vi "rad_Deploy Images with Progress_FB.vi"(6 "Deployment Notifiers":T1[](array[typedef]), 7 "temp folder":path, 8 "error in (no error)":errorcluster, 9 "Target Config Options in":T4={"NumInBatch"=0, "Target Config Operation"=enum."No Config", "Target Name"="", "Increment Static IPs"=FALSE, "Change Target Name"=FALSE, "Primary NIC"={"MAC address"="", "IP Address Request Mode"=2, "IP address"="", "Subnet mask"="", "Gateway"="", "DNS server"=""}} {"Primary NIC"."IP Address Request Mode" items=["Static"=1, "DHCP/Link-Local"=2, "Link-Local Only"=4, "DHCP Only"=8]}, 10 "RT Deployment Targets in":T2[](array[typedef]) {"Primary NIC"."IP Address Request Mode" items=["Static"=1, "DHCP/Link-Local"=2, "Link-Local Only"=4, "DHCP Only"=8]}, 11 "image path":path) -> (0 "error out":errorcluster, 1 "Target Config Options out":T4={"NumInBatch"=0, "Target Config Operation"=enum."No Config", "Target Name"="", "Increment Static IPs"=FALSE, "Change Target Name"=FALSE, "Primary NIC"={"MAC address"="", "IP Address Request Mode"=2, "IP address"="", "Subnet mask"="", "Gateway"="", "DNS server"=""}} {"Primary NIC"."IP Address Request Mode" items=["Static"=1, "DHCP/Link-Local"=2, "Link-Local Only"=4, "DHCP Only"=8]}, 2 "Error Occurred":bool[](array[boolean]))   [LabVIEW 2015]
uses:
  TypeDefs/rad_Target Configuration Settings.ctl
  TypeDefs/rad_Target Configuration Operations.ctl
  Targets/TypeDefs/rad_Target Network Settings.ctl
  Targets/TypeDefs/rad_Target Information.ctl
  TypeDefs/rad_Application Image Properties.ctl
  TypeDefs/rad_FPGA Properties.ctl
  TypeDefs/rad_FPGA Flash Properties.ctl
  TypeDefs/rad_Deployment Notifiers.ctl
  TypeDefs/rad_Deployment Status Data Type.ctl
  TypeDefs/rad_Deployment Progress Data Type.ctl
  Targets/TypeDefs/rad_Initialize Access Types.ctl
  <vilib>/nisyscfg/Close (System).vi
  <vilib>/nisyscfg/Set System Image (Folder).vi
  <vilib>/nisyscfg/nisyscfg.lvlib
panel:
  out "AppImage Properties.Model":string
  in  "State Variables":T10={"INI Modified"=FALSE, "Target Config. Options"={"NumInBatch"=0, "Target Config Operation"=enum."No Config", "Target Name"="", "Increment Static IPs"=FALSE, "Change Target Name"=FALSE, "Primary NIC"={"MAC address"="", "IP Address Request Mode"=2, "IP address"="", "Subnet mask"="", "Gateway"="", "DNS server"=""}}, "RT Deployment Targets"=[], "AppImage Properties"={"Name"="", "Version"="", "Time"=timestamp(0 s since 1904-01-01), "Description"="", "Key"="", "Chassis"="", "FPGA Properties"=[], "Model"="", "Retrieve"=[], "Deploy"=[], "Installed Software"=[]}, "Deployment Notifiers"=[], "Post-deployment access"=enum."Admin unless unlocked"} {"RT Deployment Targets"."Primary NIC"."IP Address Request Mode" items=["Static"=1, "DHCP/Link-Local"=2, "Link-Local Only"=4, "DHCP Only"=8]; "Target Config. Options"."Primary NIC"."IP Address Request Mode" items=["Static"=1, "DHCP/Link-Local"=2, "Link-Local Only"=4, "DHCP Only"=8]}
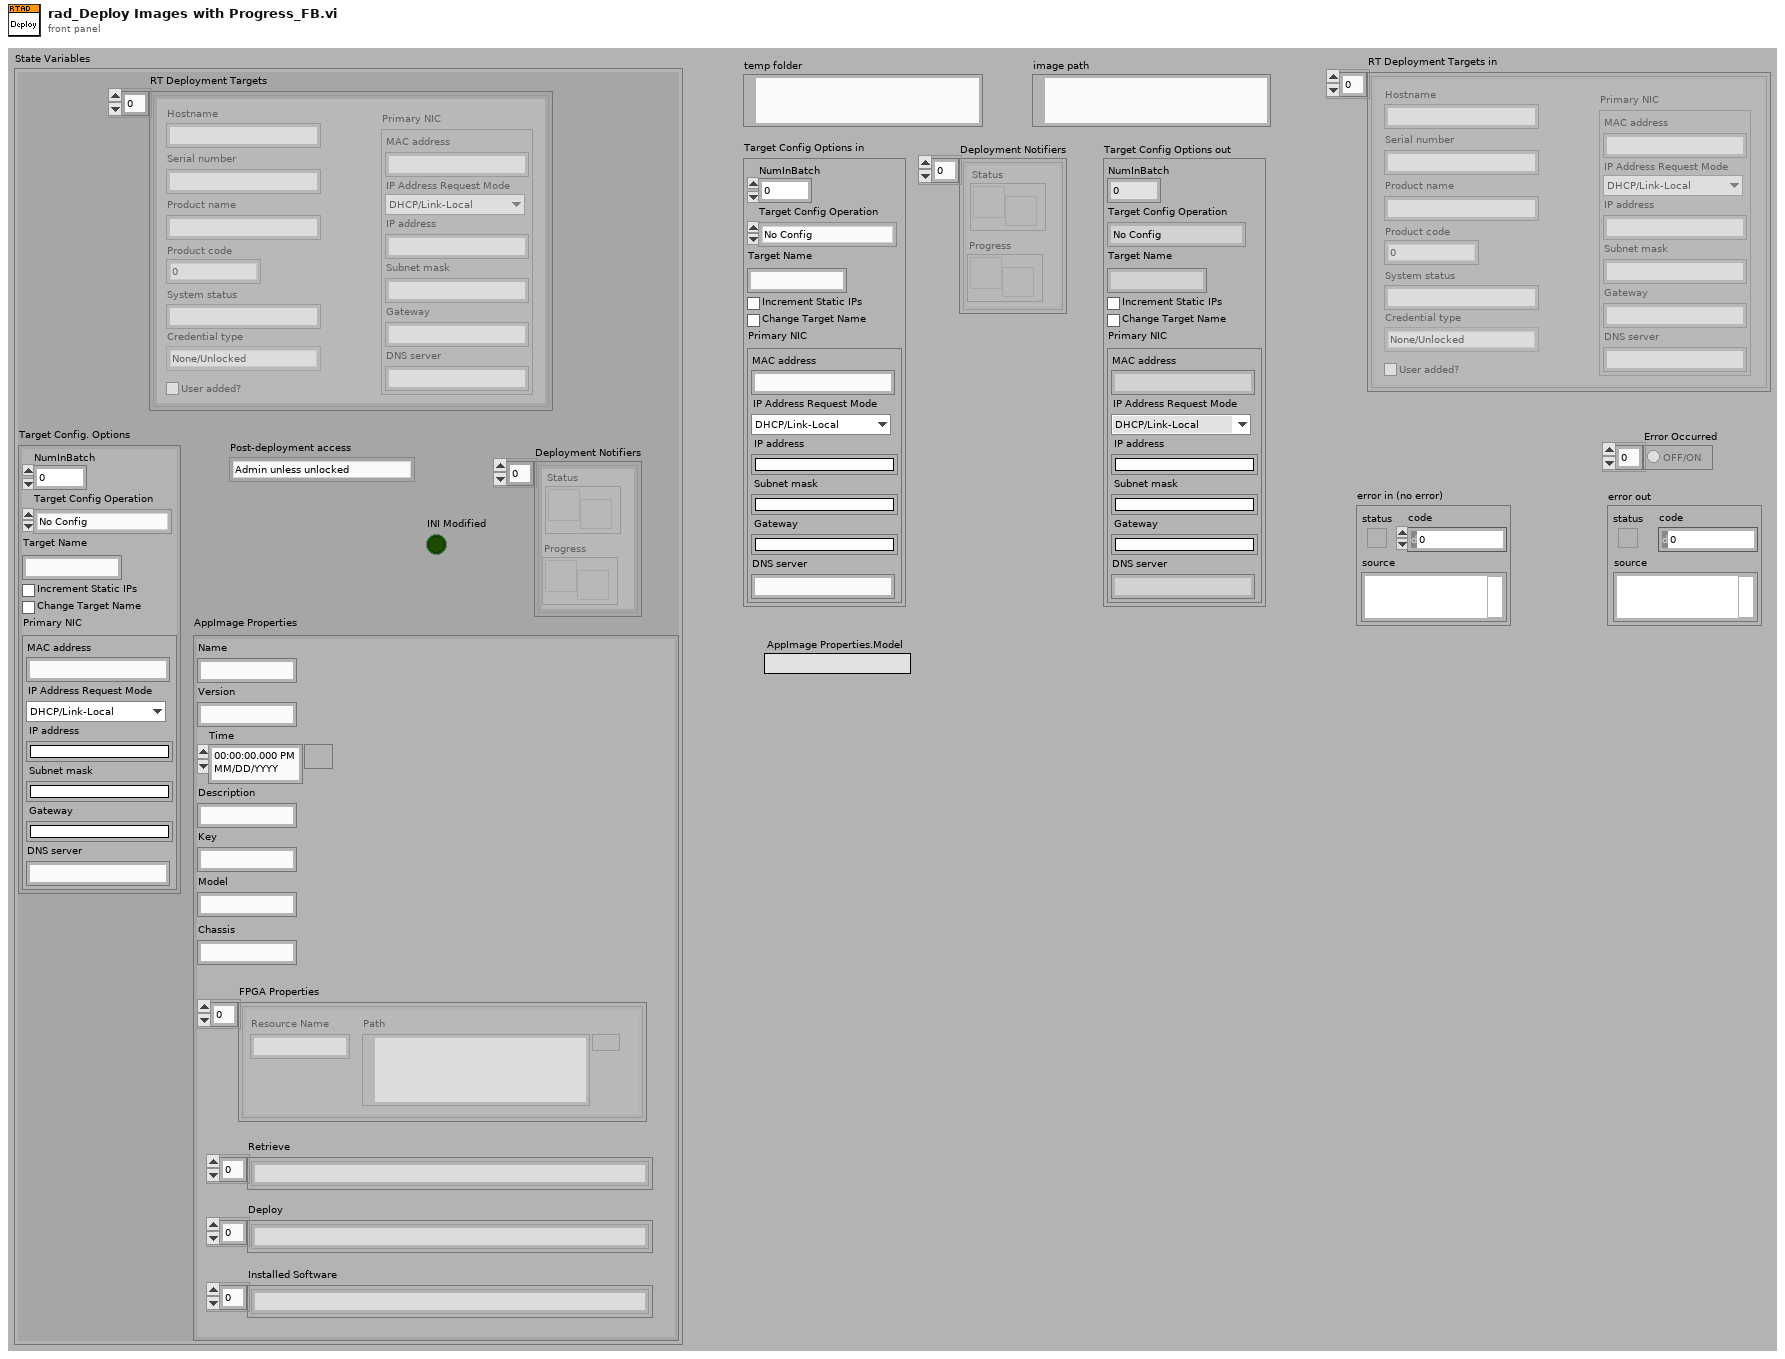
[diagram p1: front panel]
types:
  T1 = typedef "rad_Deployment Notifiers.ctl" = cluster{"Status":refnum<notifier>, "Progress":refnum<notifier>}
  T2 = typedef "rad_Target Information.ctl" = cluster{"Hostname":string, "Serial number":string, "Product name":string, "Product code":i32, "System status":string, "Credential type":enum16{"None/Unlocked", "FTP Password", "NIAuth Credentials"}, "User added?":bool, "Primary NIC":T3}
  T3 = typedef "rad_Target Network Settings.ctl" = cluster{"MAC address":string, "IP Address Request Mode":i32, "IP address":string, "Subnet mask":string, "Gateway":string, "DNS server":string}
  T4 = typedef "rad_Target Configuration Settings.ctl" = cluster{"NumInBatch":u32, "Target Config Operation":T5, "Target Name":string, "Increment Static IPs":bool, "Change Target Name":bool, "Primary NIC":T3}
  T5 = typedef "rad_Target Configuration Operations.ctl" = enum8{"No Config", "Image Config", "Static Config"}
  T6 = typedef "rad_Application Image Properties.ctl" = cluster{"Name":string, "Version":string, "Time":timestamp, "Description":string, "Key":string, "Chassis":string, "FPGA Properties":T7, "Model":string, "Retrieve":string[], "Deploy":string[], "Installed Software":string[]}
  T7 = typedef "rad_FPGA Properties.ctl" = T8[]
  T8 = typedef "rad_FPGA Flash Properties.ctl" = cluster{"Resource Name":string, "Path":path}
  T9 = typedef "rad_Initialize Access Types.ctl" = enum16{"Anonymous read-only", "Admin unless unlocked", "Admin always"}
  T10 = cluster{"INI Modified":bool, "Target Config. Options":T4, "RT Deployment Targets":T2[], "AppImage Properties":T6, "Deployment Notifiers":T1[], "Post-deployment access":T9}
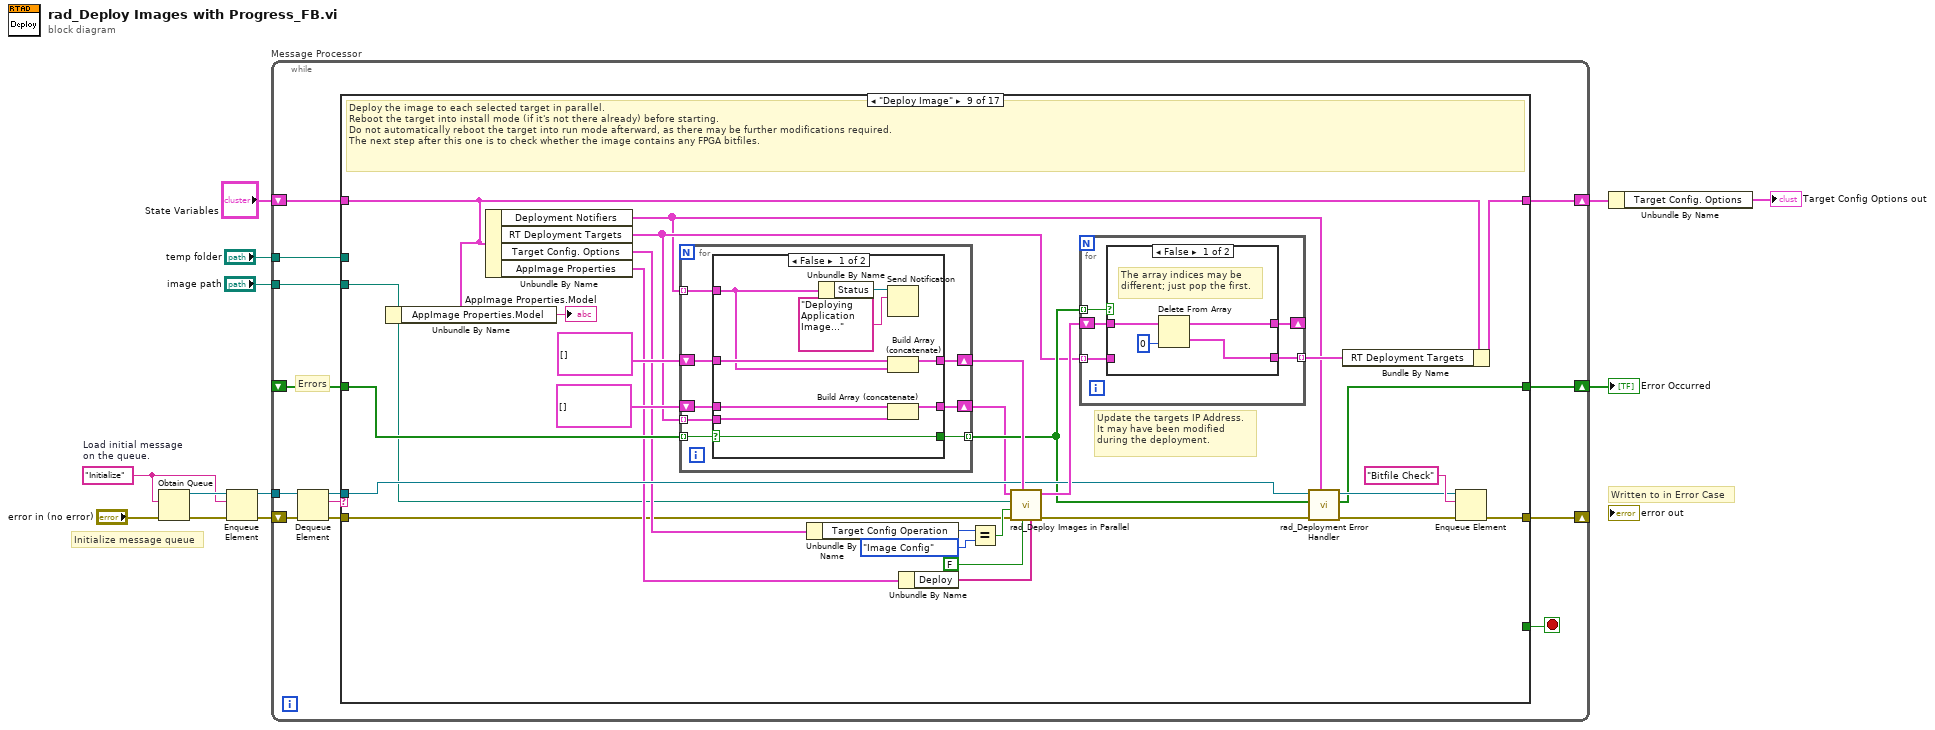
[diagram p0: block diagram]
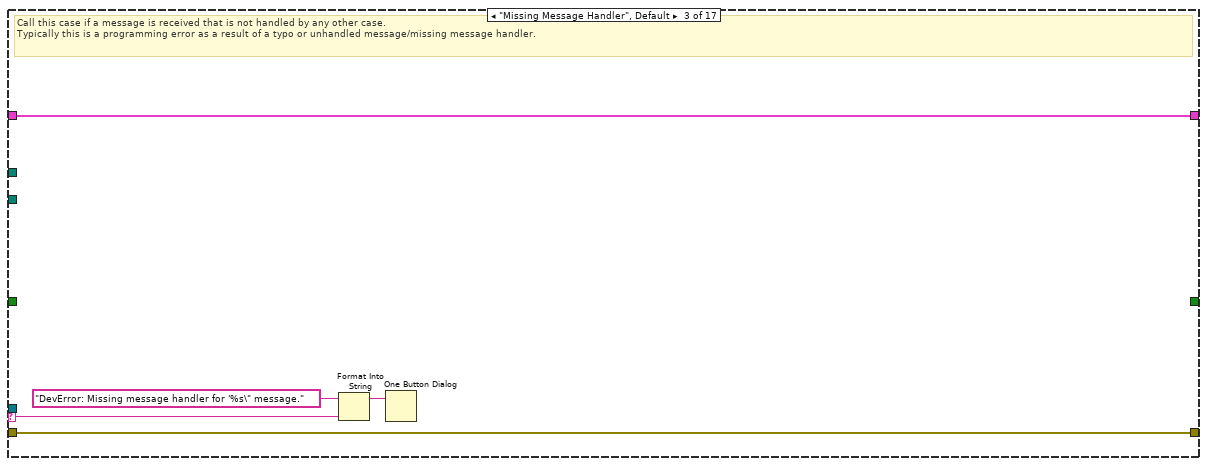
[diagram p4: hidden frame]
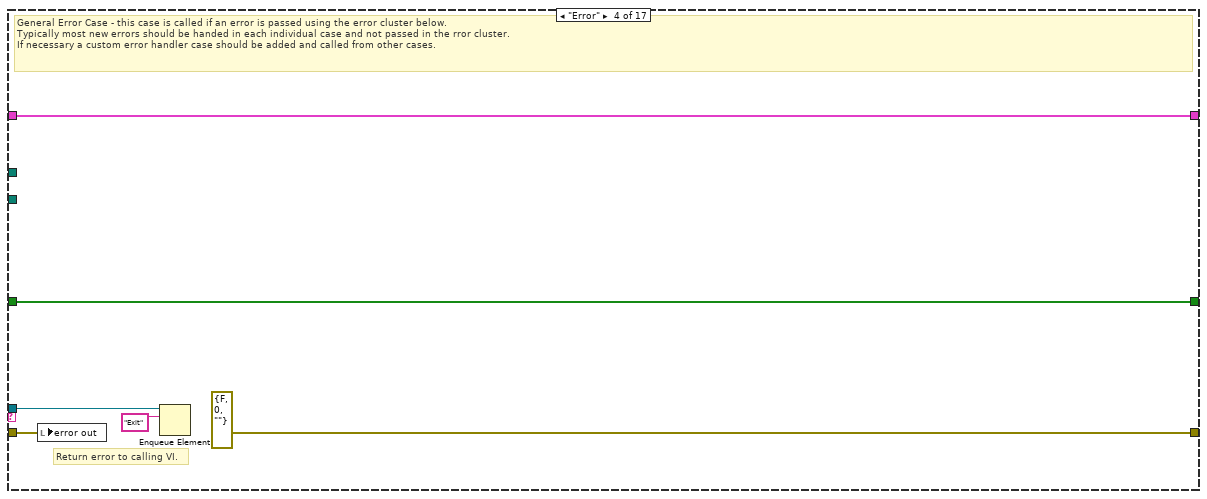
[diagram p5: hidden frame]
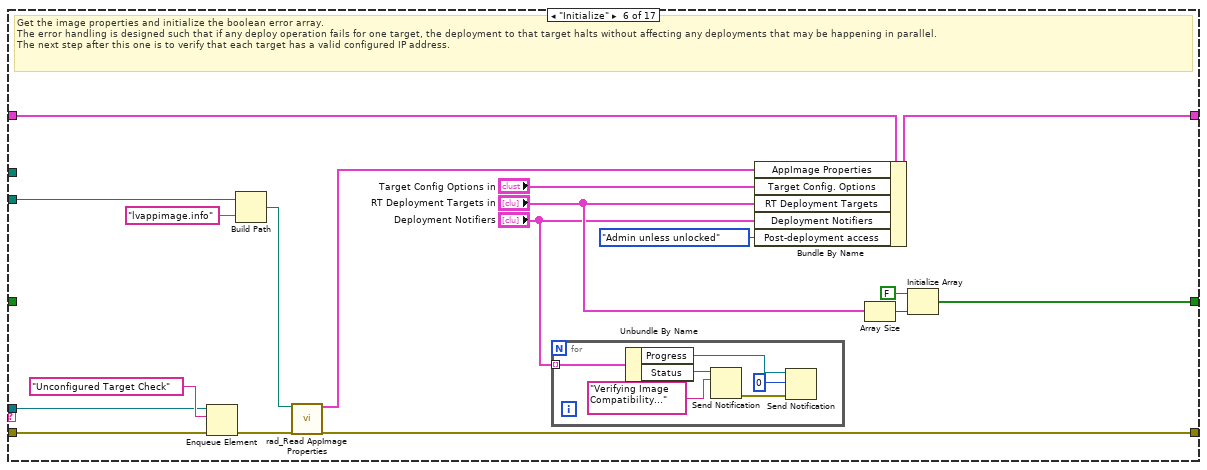
[diagram p7: hidden frame]
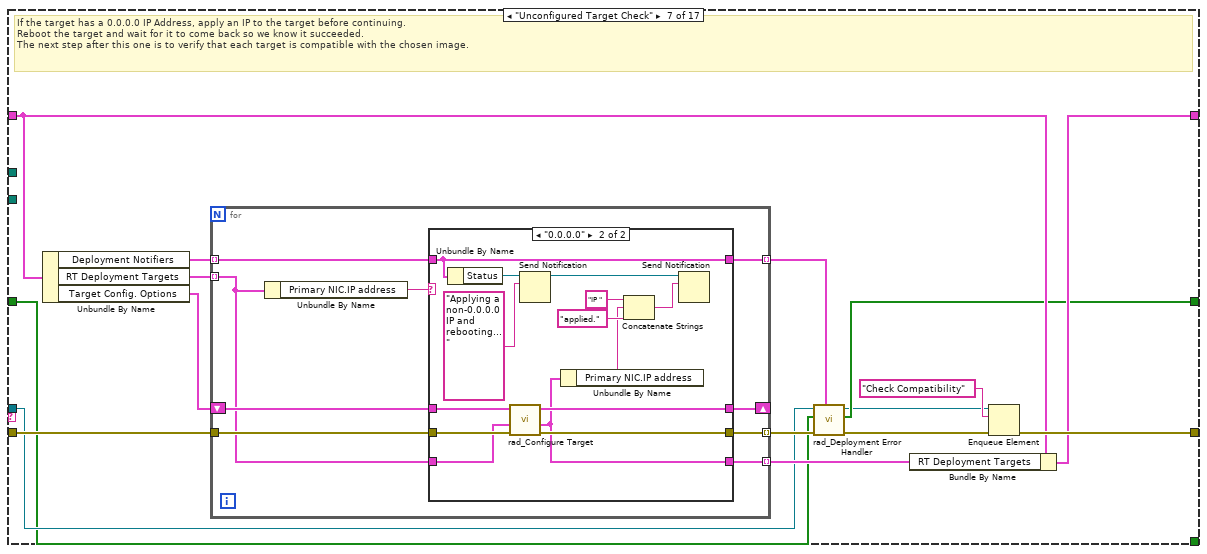
[diagram p8: hidden frame]
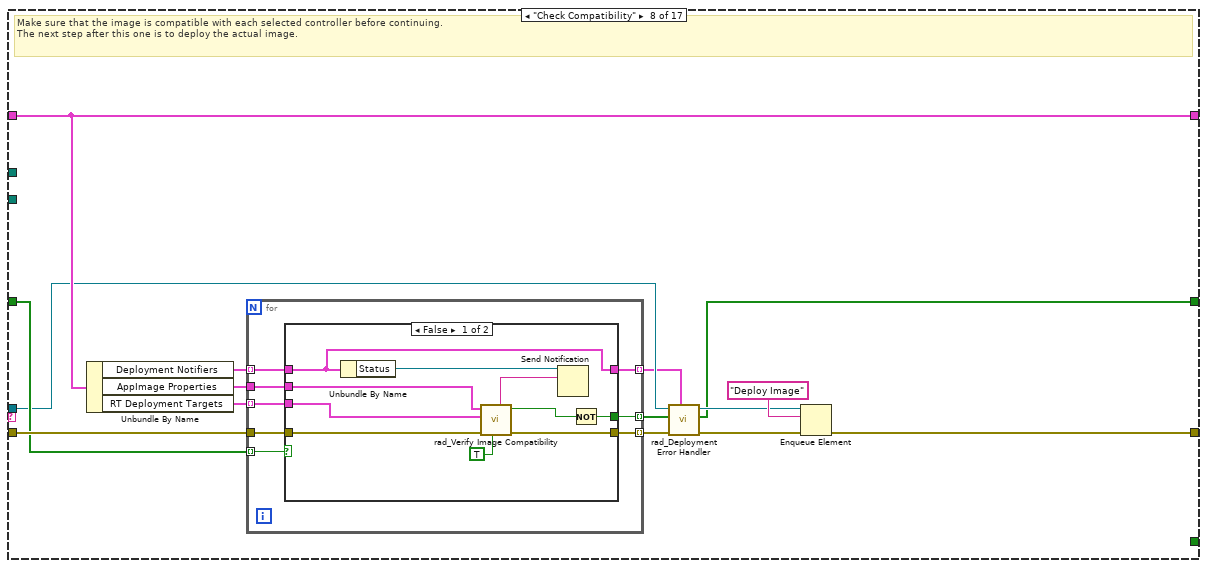
[diagram p10: hidden frame]
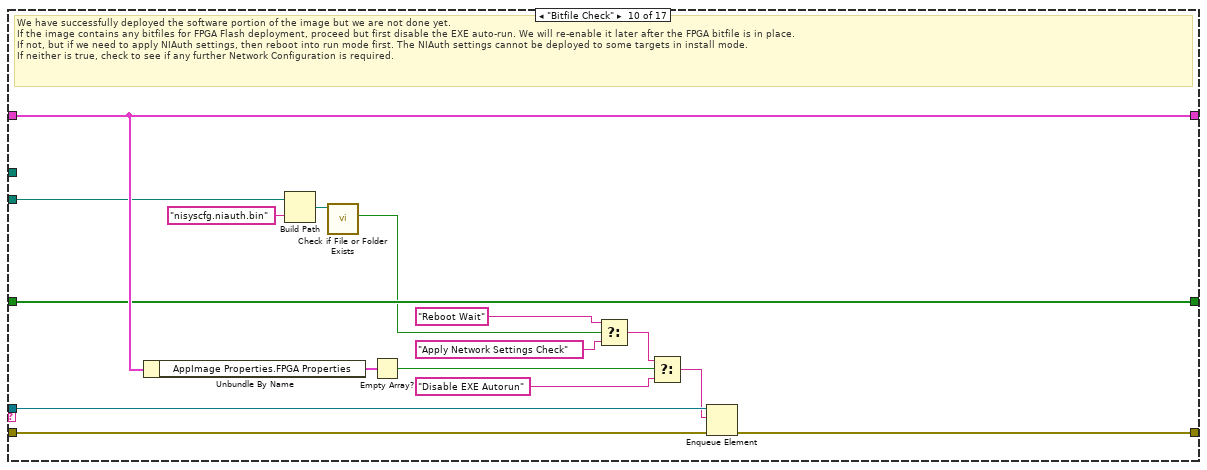
[diagram p14: hidden frame]
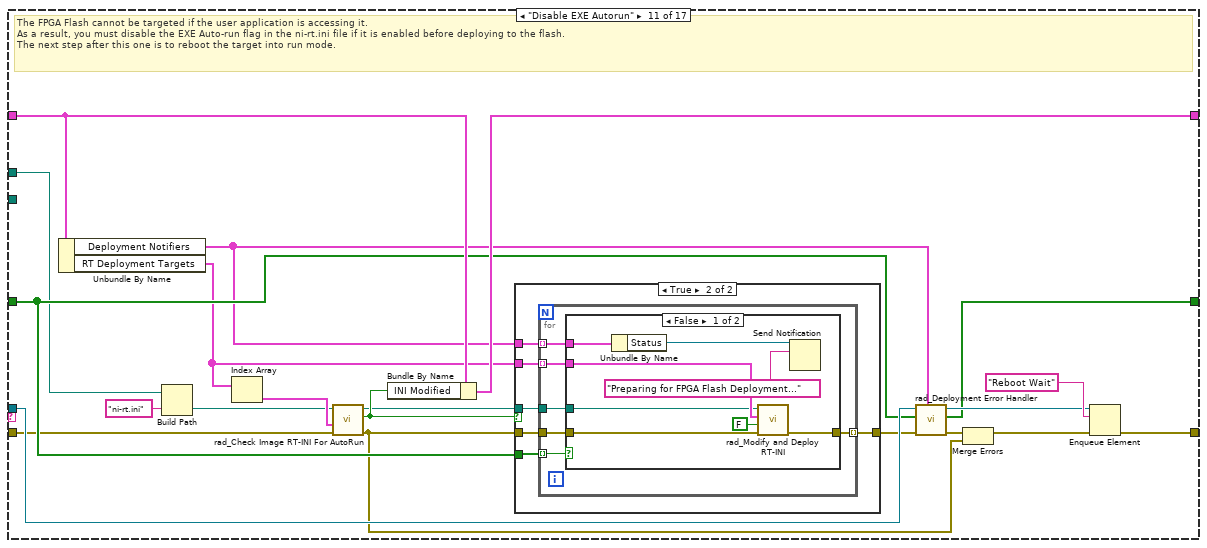
[diagram p15: hidden frame]
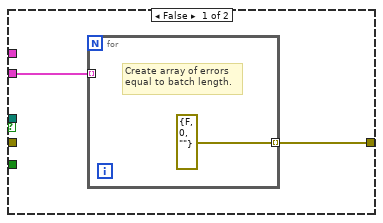
[diagram p16: hidden frame]
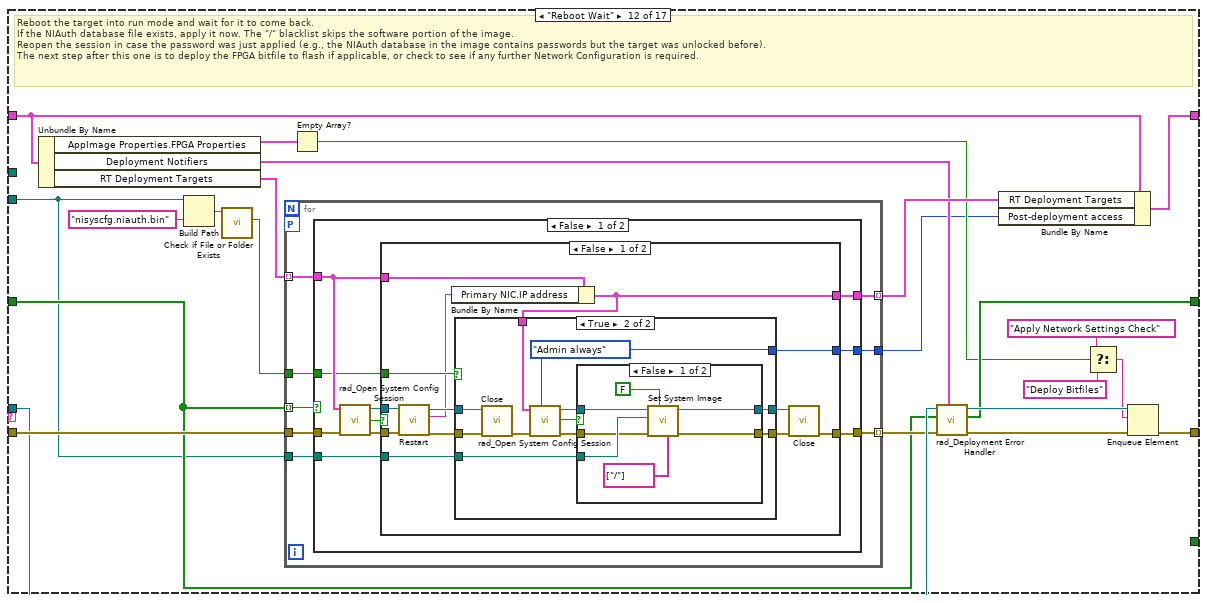
[diagram p18: hidden frame]
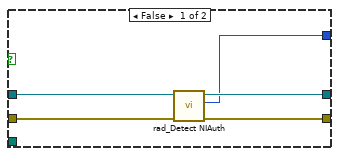
[diagram p19: hidden frame]
diagram:
  w1 = "Initialize"  # Load initial message on the queue.
  # "Written to in Error Case"
  # "Initialize message queue"
  n1 = Obtain Queue(element data type=w1, error in (no error)="error in (no error)") -> (queue out=w12:refnum<queue>, error out=w3:errorcluster)  [unwired: 3 in, 1 out]
  n2 = Enqueue Element(queue=w12, element=w1, error in (no error)=w3) -> (queue out=w4:refnum<queue>, error out=w2:errorcluster)  [unwired: 1 in, 1 out]
  n3 = while "Message Processor" {
    shift-left: w2 -> [w21]
    shift-right: [w14] -> _
    tunnel: w4 -> [w22]
    shift-left: "State Variables" -> [w25]
    shift-right: [w24] -> w9
    tunnel: "temp folder" -> [w18]
    tunnel: "image path" -> [w17]
    shift-right: [w15] -> w5
    shift-left: _ -> [w16]
    stop <- w13 stop-if-true
    # "Errors"
    n4 = Dequeue Element(queue=w22, error in (no error)=w21) -> (queue out=w23:refnum<queue>, element=w19:string, error out=w20:errorcluster)  [unwired: 1 in, 1 out]
    n5 = case shown="\"Deploy Image\"" w19 {
      selector: w19 -> [_ _ w33 _ _ _ _ _ _ _ _ _ _ _ _ _ _]
      tunnel: [w27 w30 w35 w41 w43 w60 w80 w124 w168 w220 w240 w285 w373 w413 w442 w489 w513] -> w24
      tunnel: w25 -> [w27 w30 w35 w41 w43 w61 w79 w124 w148 w220 w241 w287 w373 w413 w440 w489 w513]
      tunnel: w23 -> [_ _ _ w40 _ w45 w70 w117 w166 w221 w239 w283 w367 w410 w433 w496 w515]
      tunnel: w20 -> [w26 w29 w34 w37 w42 w50 w83 w119 w149 w219 w225 w288 w356 w401 w441 w498 w516]
      tunnel: [w26 w29 w34 errorcluster {"status"=FALSE, "code"=0, "source"=""} ("error out") w42 w51 w82 w125 w175 w222 w243 w290 w374 w412 w446 w500 w514] -> w14
      tunnel: w18 -> [_ _ _ _ _ _ _ _ _ _ w226 _ _ w402 _ _ _]
      tunnel: w17 -> [_ _ _ _ _ w49 _ _ w150 w214 _ w273 w355 _ _ _ _]
      tunnel: [_ w28 _ w36 _ w56 w74 w112 w161 w218 w236 w281 w366 w408 w431 w494 w511] -> w15
      tunnel: w16 -> [_ w28 _ w36 _ _ w68 w118 w173 w218 w233 w278 w362 w406 w426 w491 w511]
      tunnel: [_ _ _ _ _ _ _ _ _ _ _ _ _ _ _ _ TRUE] -> w13
      frame "---------- Framework Operations ----------" {
        # "Dummy case to add a seperator in the Case Structure menu."
      }
      frame "", "Idle" {
        # "Idle Case - this case is called after a Timeout on the Get Next Message from Queue VI, if no new messages are present on the queue.\nThis case can be used for housekeeping tasks such as updating the UI."
      }
      frame "Missing Message Handler", Default {
        # "Call this case if a message is received that is not handled by any other case.\nTypically this is a programming error as a result of a typo or unhandled message/missing message handler."
        n6 = Format Into String(format string="DevError: Missing message handler for '%s\" message." ("message"), w33) -> (resulting string=w31:string)  [unwired: 2 in, 1 out]
        n7 = One Button Dialog(message=w31) -> ()  [unwired: 2 out]
      }
      frame "Error" {
        # "Return error to calling VI."
        # "General Error Case - this case is called if an error is passed using the error cluster below.\nTypically most new errors should be handed in each individual case and not passed in the rror cluster.\nIf necessary a custom error handler case should be added and called from other cases."
        n8 = local write "error out"(w37) -> ()
        n9 = Enqueue Element(queue=w40, element="Exit") -> ()  [unwired: 2 in, 3 out]
      }
      frame "----------Application Operations ----------" {
        # "Dummy case to add a seperator in the Case Structure menu."
      }
      frame "Initialize" {
        # "Get the image properties and initialize the boolean error array. \nThe error handling is designed such that if any deploy operation fails for one target, the deployment to that target halts without affecting any deployments that may be happening in parallel. \nThe next step after this one is to verify that each target has a valid configured IP address."
        n10 = Enqueue Element(queue=w45, element="Unconfigured Target Check", error in (no error)=w50) -> (error out=w47:errorcluster)  [unwired: 1 in, 2 out]
        n11 = Build Path(base path=w49, name or relative path="lvappimage.info") -> (appended path=w52:path)
        n12 = call "rad_Read AppImage Properties.vi"("AppImage Properties Path"=w52, "error in (no error)"=w47) -> ("AppImage Properties"=w48:T6, "error out"=w51:errorcluster)  [unwired: 12 in, 4 out]
        n13 = for {
          tunnel: "Deployment Notifiers" -> [w66] mode=indexing
          n14 = Unbundle By Name(w66) -> ("Progress"=w64:refnum<notifier>, "Status"=w65:refnum<notifier>)
          n15 = Send Notification(notification="Verifying Image Compatibility...", notifier=w65) -> (error out=w63:errorcluster)  [unwired: 1 in, 1 out]
          n16 = Send Notification(notification=0, notifier=w64, error in (no error)=w63) -> ()  [unwired: 2 out]
        }
        n17 = Bundle By Name(cluster=w61, "AppImage Properties"=w48, "Target Config. Options"="Target Config Options in", "RT Deployment Targets"="RT Deployment Targets in", "Deployment Notifiers"="Deployment Notifiers", "Post-deployment access"=rad_Initialize_Access_Types."Admin unless unlocked") -> (w60:T10)
        n18 = Array Size(array="RT Deployment Targets in") -> (size(s)=w57:i32)
        n19 = Initialize Array(FALSE, w57) -> (w56:bool[])
      }
      frame "Unconfigured Target Check" {
        # "If the target has a 0.0.0.0 IP Address, apply an IP to the target before continuing. \nReboot the target and wait for it to come back so we know it succeeded. \nThe next step after this one is to verify that each target is compatible with the chosen image."
        n20 = Unbundle By Name(w79) -> ("Deployment Notifiers"=w78:T1[], "RT Deployment Targets"=w77:T2[], "Target Config. Options"=w76:T4)
        n21 = for {
          tunnel: w83 -> [w90]
          tunnel: [w92] -> w73 mode=indexing
          tunnel: w78 -> [w88] mode=indexing
          tunnel: w77 -> [w87] mode=indexing
          shift-right: [w89] -> _
          shift-left: w76 -> [w91]
          tunnel: [w86] -> w75 mode=indexing
          tunnel: [w85] -> w71 mode=indexing
          n22 = Unbundle By Name(w87) -> ("Primary NIC.IP address"=w84:string)
          n23 = case shown="\"0.0.0.0\"" w84 {
            tunnel: [w96 w102] -> w92
            tunnel: w91 -> [w94 w110]
            tunnel: w90 -> [w96 w103]
            tunnel: [w94 w109] -> w89
            tunnel: w88 -> [w93 w100]
            tunnel: w87 -> [w95 w99]
            tunnel: [w95 w98] -> w86
            tunnel: [w93 w100] -> w85
            frame Default {
            }
            frame "0.0.0.0" {
              n24 = Unbundle By Name(w100) -> ("Status"=w101:refnum<notifier>)
              n25 = call "rad_Configure Target.vi"("error in (no error)"=w103, "Target settings in"=w99, "Target Config Options in"=w110) -> ("error out"=w102:errorcluster, "Target settings out"=w98:T2, "Target Config Options out"=w109:T4)  [unwired: 6 in]
              n26 = Send Notification(notification="Applying a non-0.0.0.0 IP and rebooting...", notifier=w101) -> (notifier out=w107:refnum<notifier>)  [unwired: 1 in, 1 out]
              n27 = Unbundle By Name(w98) -> ("Primary NIC.IP address"=w97:string)
              n28 = Concatenate Strings("IP " ("notification"), w97, "applied." ("string")) -> (w104:string)
              n29 = Send Notification(notification=w104, notifier=w107) -> ()  [unwired: 1 in, 2 out]
            }
          }
        }
        n30 = call "rad_Deployment Error Handler.vi"("Deployment Notifiers"=w71, "error in (no error)"=w73, "Error Occurred"=w68, "Queue in"=w70) -> ("error out"=w72:errorcluster, "Error Occurred"=w74:bool[], "Queue out"=w69:refnum<queue>)  [unwired: 5 in]
        n31 = Bundle By Name(cluster=w79, "RT Deployment Targets"=w75) -> (w80:T10)
        n32 = Enqueue Element(queue=w69, element="Check Compatibility" ("Message Name"), error in (no error)=w72) -> (error out=w82:errorcluster)  [unwired: 1 in, 2 out]
      }
      frame "Check Compatibility" {
        # "Make sure that the image is compatible with each selected controller before continuing.\nThe next step after this one is to deploy the actual image."
        n33 = Unbundle By Name(w124) -> ("Deployment Notifiers"=w121:T1[], "AppImage Properties"=w120:T6, "RT Deployment Targets"=w122:T2[])
        n34 = for {
          tunnel: w122 -> [w131] mode=indexing
          tunnel: w121 -> [w129] mode=indexing
          tunnel: w120 -> [w133]
          tunnel: w119 -> [w132]
          tunnel: w118 -> [w130] mode=indexing
          tunnel: [w128] -> w115 mode=indexing
          tunnel: [w127] -> w116 mode=indexing
          tunnel: [w126] -> w114 mode=indexing
          n35 = case shown="False" w130 {
            selector: w130 -> [_ w146]
            tunnel: w133 -> [w143 _]
            tunnel: w132 -> [w142 w145]
            tunnel: w131 -> [w134 _]
            tunnel: w129 -> [w136 w144]
            tunnel: [w138 w146] -> w128
            tunnel: [w140 w145] -> w127
            tunnel: [w136 w144] -> w126
            frame False {
              n36 = Unbundle By Name(w136) -> ("Status"=w137:refnum<notifier>)
              n37 = call "rad_Verify Image Compatibility.vi"("Require Identical Chassis?"=TRUE, "error in (no error)"=w142, "Target address"=w134, "AppImage Properties"=w143) -> ("error out"=w140:errorcluster, "Compatible?"=w139:bool, "Status message"=w135:string)  [unwired: 5 in]
              n38 = Send Notification(notification=w135, notifier=w137) -> ()  [unwired: 1 in, 2 out]
              n39 = Not(x=w139) -> (.not. x?=w138:bool)
            }
            frame True {
            }
          }
        }
        n40 = call "rad_Deployment Error Handler.vi"("Deployment Notifiers"=w114, "error in (no error)"=w116, "Error Occurred"=w115, "Queue in"=w117) -> ("error out"=w111:errorcluster, "Error Occurred"=w112:bool[], "Queue out"=w113:refnum<queue>)  [unwired: 5 in]
        n41 = Enqueue Element(queue=w113, element="Deploy Image" ("t"), error in (no error)=w111) -> (error out=w125:errorcluster)  [unwired: 1 in, 2 out]
      }
      frame "Deploy Image" {
        # "Update the targets IP Address.\nIt may have been modified\nduring the deployment."
        # "Deploy the image to each selected target in parallel. \nReboot the target into install mode (if it's not there already) before starting.\nDo not automatically reboot the target into run mode afterward, as there may be further modifications required. \nThe next step after this one is to check whether the image contains any FPGA bitfiles."
        n42 = Unbundle By Name(w148) -> ("AppImage Properties.Model"=→"AppImage Properties.Model":string)
        n43 = Unbundle By Name(w148) -> ("Deployment Notifiers"=w158:T1[], "RT Deployment Targets"=w159:T2[], "Target Config. Options"=w154:T4, "AppImage Properties"=w153:T6)
        n44 = for {
          tunnel: w158 -> [w193] mode=indexing
          tunnel: w173 -> [w194] mode=indexing
          tunnel: [w192] -> w164 mode=indexing
          tunnel: w159 -> [w191] mode=indexing
          shift-right: [w190] -> w170
          shift-left: T1[] [] ("Deployment Notifiers") -> [w189]
          shift-right: [w188] -> w151
          shift-left: T2[] [] -> [w187]
          n45 = case shown="False" w194 {
            selector: w194 -> [w202 w206]
            tunnel: w193 -> [w197 _]
            tunnel: [w202 w206] -> w192
            tunnel: w191 -> [w195 _]
            tunnel: [w201 w204] -> w190
            tunnel: w189 -> [w200 w204]
            tunnel: [w199 w205] -> w188
            tunnel: w187 -> [w198 w205]
            frame False {
              n46 = Unbundle By Name(w197) -> ("Status"=w196:refnum<notifier>)
              n47 = Send Notification(notification="Deploying Application Image...", notifier=w196) -> ()  [unwired: 1 in, 2 out]
              n48 = Build Array (concatenate)(w200, w197) -> (w201:T1[])
              n49 = Build Array (concatenate)(w198, w195) -> (w199:T2[])
            }
            frame True {
            }
          }
        }
        n50 = Unbundle By Name(w154) -> ("Target Config Operation"=w157:T5)
        n51 = Unbundle By Name(w153) -> ("Deploy"=w152:string[])
        n52 = Equal?(x=w157, y=rad_Target_Configuration_Operations."Image Config" ("x")) -> (x = y?=w155:bool)
        n53 = call "rad_Deploy Images in Parallel.vi"("Deploy"=w152, "restart after imaging (T)"=FALSE ("restart after imaging? (T)"), "Deployment Notifiers"=w170, "error in (no error)"=w149, "apply primary NIC from image (F)"=w155, "image file path in"=w150, "Target addresses in"=w151) -> ("Errors Out"=w165:errorcluster[], "Target addresses out"=w169:T2[])  [unwired: 2 in, 1 out]
        n54 = for {
          tunnel: w164 -> [w180] mode=indexing
          tunnel: w159 -> [w178] mode=indexing
          shift-right: [w176] -> _
          shift-left: w169 -> [w179]
          tunnel: [w177] -> w167 mode=indexing
          n55 = case shown="False" w180 {
            tunnel: w179 -> [w184 w186]
            tunnel: w178 -> [_ w185]
            tunnel: [w182 w185] -> w177
            tunnel: [w183 w186] -> w176
            frame False {
              # "The array indices may be\ndifferent; just pop the first."
              n56 = Delete From Array(array=w184, index=0) -> (deleted portion=w182:T2, array with subset deleted=w183:T2[])  [unwired: 1 in]
            }
            frame True {
              # "An error happened earlier,\nso keep the existing address."
            }
          }
        }
        n57 = call "rad_Deployment Error Handler.vi"("Deployment Notifiers"=w158, "error in (no error)"=w165, "Error Occurred"=w164, "Queue in"=w166) -> ("error out"=w162:errorcluster, "Error Occurred"=w161:bool[], "Queue out"=w163:refnum<queue>)  [unwired: 5 in]
        n58 = Bundle By Name(cluster=w148, "RT Deployment Targets"=w167) -> (w168:T10)
        n59 = Enqueue Element(queue=w163, element="Bitfile Check" ("Message Name"), error in (no error)=w162) -> (error out=w175:errorcluster)  [unwired: 1 in, 2 out]
      }
      frame "Bitfile Check" {
        # "We have successfully deployed the software portion of the image but we are not done yet.\nIf the image contains any bitfiles for FPGA Flash deployment, proceed but first disable the EXE auto-run. We will re-enable it later after the FPGA bitfile is in place.\nIf not, but if we need to apply NIAuth settings, then reboot into run mode first. The NIAuth settings cannot be deployed to some targets in install mode.\nIf neither is true, check to see if any further Network Configuration is required."
        n60 = Unbundle By Name(w220) -> ("AppImage Properties.FPGA Properties"=w217:T7)
        n61 = Build Path(base path=w214, name or relative path="nisyscfg.niauth.bin") -> (appended path=w212:path)
        n62 = call <vilib>:"Check if File or Folder Exists.vi"("path"=w212) -> ("file or folder exists?"=w209:bool)  [unwired: 8 in, 2 out]
        n63 = Empty Array?(array=w217) -> (empty?=w215:bool)
        n64 = Select(t="Reboot Wait" ("Title"), s=w209, f="Apply Network Settings Check" ("Title")) -> (s? t:f=w210:string)
        n65 = Select(t=w210, s=w215, f="Disable EXE Autorun" ("Title")) -> (s? t:f=w211:string)
        n66 = Enqueue Element(queue=w221, element=w211, error in (no error)=w219) -> (error out=w222:errorcluster)  [unwired: 1 in, 2 out]
      }
      frame "Disable EXE Autorun" {
        # "The FPGA Flash cannot be targeted if the user application is accessing it.\nAs a result, you must disable the EXE Auto-run flag in the ni-rt.ini file if it is enabled before deploying to the flash.\nThe next step after this one is to reboot the target into run mode."
        n67 = Unbundle By Name(w241) -> ("Deployment Notifiers"=w232:T1[], "RT Deployment Targets"=w231:T2[])
        n68 = Build Path(base path=w226, name or relative path="ni-rt.ini") -> (appended path=w224:path)
        n69 = Index Array(array=w231) -> (element=w227:T2)  [unwired: 1 in]
        n70 = call "rad_Check Image RT-INI For AutoRun.vi"("error in (no error)"=w225, "target settings"=w227, "temp folder"=w224) -> ("error out"=w230:errorcluster, "Run at Startup?"=w229:bool, "temp folder out"=w228:path)  [unwired: 6 in]
        n71 = Bundle By Name(cluster=w241, "INI Modified"=w229) -> (w240:T10)
        n72 = case shown="True" w229 {
          tunnel: [w244 w251] -> w237
          tunnel: w230 -> [_ w252]
          tunnel: w231 -> [w245 w250]
          tunnel: w233 -> [_ w249]
          tunnel: w232 -> [_ w248]
          tunnel: w228 -> [_ w247]
          frame False {
            n73 = for {
              tunnel: w245 -> [_] mode=indexing
              tunnel: [errorcluster {"status"=FALSE, "code"=0, "source"=""} ("error out")] -> w244 mode=indexing
              # "Create array of errors\nequal to batch length."
            }
          }
          frame True {
            n74 = for {
              tunnel: w252 -> [w258]
              tunnel: [w257] -> w251 mode=indexing
              tunnel: w250 -> [w256] mode=indexing
              tunnel: w249 -> [w255] mode=indexing
              tunnel: w248 -> [w254] mode=indexing
              tunnel: w247 -> [w253]
              n75 = case shown="False" w255 {
                tunnel: w258 -> [w260 w267]
                tunnel: [w265 w267] -> w257
                tunnel: w256 -> [w261 _]
                tunnel: w254 -> [w263 _]
                tunnel: w253 -> [w259 _]
                frame False {
                  n76 = Unbundle By Name(w263) -> ("Status"=w262:refnum<notifier>)
                  n77 = call "rad_Modify and Deploy RT-INI.vi"("error in (no error)"=w260, "Run at Startup?"=FALSE, "Target settings"=w261, "temp folder"=w259) -> ("error out"=w265:errorcluster)  [unwired: 7 in]
                  n78 = Send Notification(notification="Preparing for FPGA Flash Deployment...", notifier=w262) -> ()  [unwired: 1 in, 2 out]
                }
                frame True {
                }
              }
            }
          }
        }
        n79 = call "rad_Deployment Error Handler.vi"("Deployment Notifiers"=w232, "error in (no error)"=w237, "Error Occurred"=w233, "Queue in"=w239) -> ("error out"=w235:errorcluster, "Error Occurred"=w236:bool[], "Queue out"=w238:refnum<queue>)  [unwired: 5 in]
        n80 = Merge Errors(w235, w230) -> (w234:errorcluster)
        n81 = Enqueue Element(queue=w238, element="Reboot Wait" ("Message Name"), error in (no error)=w234) -> (error out=w243:errorcluster)  [unwired: 1 in, 2 out]
      }
      frame "Reboot Wait" {
        # "Reboot the target into run mode and wait for it to come back.\nIf the NIAuth database file exists, apply it now. The \"/\" blacklist skips the software portion of the image.\nReopen the session in case the password was just applied (e.g., the NIAuth database in the image contains passwords but the target was unlocked before).\nThe next step after this one is to deploy the FPGA bitfile to flash if applicable, or check to see if any further Network Configuration is required."
        n82 = Unbundle By Name(w287) -> ("AppImage Properties.FPGA Properties"=w277:T7, "Deployment Notifiers"=w284:T1[], "RT Deployment Targets"=w289:T2[])
        n83 = Build Path(base path=w273, name or relative path="nisyscfg.niauth.bin") -> (appended path=w275:path)
        n84 = call <vilib>:"Check if File or Folder Exists.vi"("path"=w275) -> ("file or folder exists?"=w274:bool)  [unwired: 8 in, 2 out]
        n85 = for {
          tunnel: w289 -> [w296] mode=indexing
          tunnel: w288 -> [w298]
          tunnel: [w297] -> w279 mode=indexing
          tunnel: [w295] -> w286 mode=indexing
          tunnel: w278 -> [w294] mode=indexing
          workers-P: _ -> [_]
          tunnel: w274 -> [w293]
          tunnel: w273 -> [w292]
          tunnel: [w291] -> w268
          n86 = case shown="False" w294 {
            tunnel: w298 -> [w308 w351]
            tunnel: [w301 w351] -> w297
            tunnel: w296 -> [w304 w352]
            tunnel: [w303 w352] -> w295
            tunnel: w293 -> [w302 _]
            tunnel: w292 -> [w300 _]
            tunnel: [w299 rad_Initialize_Access_Types."Admin unless unlocked" ("Access requirement (admin unless unlocked)")] -> w291
            frame False {
              n87 = call "rad_Open System Config Session.vi"("error in (no error)"=w308, "Target settings"=w304) -> ("error out"=w305:errorcluster, "Cancelled"=w307:bool, "Session out"=w306:refnum<k21>)  [unwired: 6 in, 1 out]
              n88 = case shown="False" w307 {
                tunnel: w306 -> [w320 _]
                tunnel: w305 -> [w321 w348]
                tunnel: w304 -> [w312 w349]
                tunnel: [w310 w349] -> w303
                tunnel: w302 -> [w319 _]
                tunnel: [w314 w348] -> w301
                tunnel: w300 -> [w313 _]
                tunnel: [w309 rad_Initialize_Access_Types."Admin unless unlocked" ("Access requirement (admin unless unlocked)")] -> w299
                frame False {
                  n89 = call <vilib>:"Restart.vi"("error in (no error)"=w321, "Session in"=w320) -> ("error out"=w317:errorcluster, "New IP Address"=w311:string, "Session out"=w318:refnum<k21>)  [unwired: 7 in]
                  n90 = Bundle By Name(cluster=w312, "Primary NIC.IP address"=w311) -> (w310:T2)
                  n91 = case shown="True" w319 {
                    tunnel: w318 -> [w326 w333]
                    tunnel: w317 -> [w325 w334]
                    tunnel: [w323 w336] -> w316
                    tunnel: [w324 w337] -> w315
                    tunnel: w313 -> [_ w335]
                    tunnel: [w322 w328] -> w309
                    tunnel: w310 -> [_ w327]
                    frame False {
                      n92 = call "rad_Detect NIAuth.vi"("error in (no error)"=w325, "Session in"=w326) -> ("error out"=w324:errorcluster, "Post-deployment access"=w322:T9, "Session out"=w323:refnum<k21>)  [unwired: 7 in]
                    }
                    frame True {
                      w328 = rad_Initialize_Access_Types."Admin always" ("Access requirement (admin unless unlocked)")
                      n93 = call-poly <vilib>:"Close.vi"("error in (no error)"=w334, "Session in"=w333) -> ("error out"=w332:errorcluster)  [unwired: 9 in]
                      n94 = call "rad_Open System Config Session.vi"("Access requirement (admin unless unlocked)"=w328, "error in (no error)"=w332, "Target settings"=w327) -> ("error out"=w329:errorcluster, "Cancelled"=w331:bool, "Session out"=w330:refnum<k21>)  [unwired: 5 in, 1 out]
                      n95 = case shown="False" w331 {
                        tunnel: [w344 w345] -> w337
                        tunnel: [w343 w346] -> w336
                        tunnel: w335 -> [w340 _]
                        tunnel: w330 -> [w339 w346]
                        tunnel: w329 -> [w338 w345]
                        frame False {
                          n96 = call-poly <vilib>:"Set System Image.vi"("File and Directory Blacklist"=string[] ["/"], "Restart Automatically (T)"=FALSE ("restart automatically (T)"), "error in (no error)"=w338, "Source Folder"=w340, "Session in"=w339) -> ("error out"=w344:errorcluster, "Session out"=w343:refnum<k21>)  [unwired: 5 in]
                        }
                        frame True {
                        }
                      }
                    }
                  }
                  n97 = call-poly <vilib>:"Close.vi"("error in (no error)"=w315, "Session in"=w316) -> ("error out"=w314:errorcluster)  [unwired: 9 in]
                }
                frame True {
                }
              }
            }
            frame True {
            }
          }
        }
        n98 = Empty Array?(array=w277) -> (empty?=w269:bool)
        n99 = call "rad_Deployment Error Handler.vi"("Deployment Notifiers"=w284, "error in (no error)"=w279, "Error Occurred"=w278, "Queue in"=w283) -> ("error out"=w280:errorcluster, "Error Occurred"=w281:bool[], "Queue out"=w282:refnum<queue>)  [unwired: 5 in]
        n100 = Bundle By Name(cluster=w287, "RT Deployment Targets"=w286, "Post-deployment access"=w268) -> (w285:T10)
        n101 = Select(t="Apply Network Settings Check" ("Message Name"), s=w269, f="Deploy Bitfiles" ("Message Name")) -> (s? t:f=w270:string)
        n102 = Enqueue Element(queue=w282, element=w270, error in (no error)=w280) -> (error out=w290:errorcluster)  [unwired: 1 in, 2 out]
      }
      frame "Deploy Bitfiles" {
        # "We have at least one FPGA bitfile and the EXE is not running, so deploy the bitfile to flash now.\nThe next step after this one is to re-enable the EXE Autorun flag in the ni-rt.ini file if it was modified, or check to see if any further Network Configuration is required."
        n103 = Unbundle By Name(w373) -> ("Deployment Notifiers"=w354:T1[], "Post-deployment access"=w353:T9, "RT Deployment Targets"=w368:T2[], "AppImage Properties.FPGA Properties"=w360:T7, "INI Modified"=w369:bool)
        n104 = List Folder(path=w355, pattern="*.lvbitx", error in=w356) -> (filenames=w358:string[])  [unwired: 1 in, 3 out]
        n105 = for {
          tunnel: w355 -> [w377]
          tunnel: w358 -> [w376] mode=indexing
          tunnel: [w375] -> w357 mode=indexing
          n106 = Build Path(base path=w377, name or relative path=w376) -> (appended path=w375:path)
        }
        n107 = for {
          tunnel: w360 -> [w385]
          tunnel: w357 -> [w384]
          tunnel: [w383] -> w365 mode=indexing
          tunnel: w368 -> [w382] mode=indexing
          tunnel: w356 -> [w381]
          tunnel: w354 -> [w380] mode=indexing
          tunnel: w362 -> [w379] mode=indexing
          tunnel: w353 -> [w378]
          n108 = case shown="False" w379 {
            tunnel: w385 -> [w396 _]
            tunnel: w384 -> [w395 _]
            tunnel: [w391 errorcluster {"status"=FALSE, "code"=0, "source"=""} ("error out")] -> w383
            tunnel: w382 -> [w387 _]
            tunnel: w381 -> [w394 _]
            tunnel: w380 -> [w389 _]
            tunnel: w378 -> [w386 _]
            frame False {
              n109 = Unbundle By Name(w389) -> ("Status"=w388:refnum<notifier>)
              n110 = Send Notification(notification="Deploying to FPGA Flash...", notifier=w388) -> (notifier out=w392:refnum<notifier>)  [unwired: 1 in, 1 out]
              n111 = call "rad_Deploy All Bitfiles.vi"("Access requirement"=w386, "error in (no error)"=w394, "FPGA Properties"=w396, "Unzipped files"=w395, "Target settings in"=w387) -> ("error out"=w391:errorcluster)  [unwired: 6 in]
              n112 = Send Notification(notification="FPGA Flash Deployed.", notifier=w392, error in (no error)=w391) -> ()  [unwired: 2 out]
            }
            frame True {
            }
          }
        }
        n113 = call "rad_Deployment Error Handler.vi"("Deployment Notifiers"=w354, "error in (no error)"=w365, "Error Occurred"=w362, "Queue in"=w367) -> ("error out"=w364:errorcluster, "Error Occurred"=w366:bool[], "Queue out"=w361:refnum<queue>)  [unwired: 5 in]
        n114 = Select(t="Enable EXE Autorun" ("Title"), s=w369, f="Apply Network Settings Check") -> (s? t:f=w371:string)
        n115 = Merge Errors(w364, w356) -> (w363:errorcluster)
        n116 = Enqueue Element(queue=w361, element=w371, error in (no error)=w363) -> (error out=w374:errorcluster)  [unwired: 1 in, 2 out]
      }
      frame "Enable EXE Autorun" {
        # "Re-enable the startup EXE in the ni-rt.ini file if it was disabled previously.\nThe next step after this one is to check to see if any further Network Configuration is required."
        n117 = Build Path(base path=w402, name or relative path="ni-rt.ini") -> (appended path=w399:path)
        n118 = Unbundle By Name(w413) -> ("Deployment Notifiers"=w400:T1[], "RT Deployment Targets"=w403:T2[])
        n119 = for {
          tunnel: w399 -> [w418]
          tunnel: w401 -> [w417]
          tunnel: w403 -> [w415] mode=indexing
          tunnel: [w416] -> w409 mode=indexing
          tunnel: w406 -> [w414] mode=indexing
          n120 = case shown="False" w414 {
            tunnel: w418 -> [w419 _]
            tunnel: w417 -> [w420 _]
            tunnel: [w422 errorcluster {"status"=FALSE, "code"=0, "source"=""} ("error out")] -> w416
            tunnel: w415 -> [w421 _]
            frame False {
              n121 = call "rad_Modify and Deploy RT-INI.vi"("error in (no error)"=w420, "Run at Startup?"=TRUE, "Target settings"=w421, "temp folder"=w419) -> ("error out"=w422:errorcluster)  [unwired: 7 in]
            }
            frame True {
            }
          }
        }
        n122 = call "rad_Deployment Error Handler.vi"("Deployment Notifiers"=w400, "error in (no error)"=w409, "Error Occurred"=w406, "Queue in"=w410) -> ("error out"=w405:errorcluster, "Error Occurred"=w408:bool[], "Queue out"=w407:refnum<queue>)  [unwired: 5 in]
        n123 = Merge Errors(w405, w401) -> (w404:errorcluster)
        n124 = Enqueue Element(queue=w407, element="Apply Network Settings Check" ("Message Name"), error in (no error)=w404) -> (error out=w412:errorcluster)  [unwired: 1 in, 2 out]
      }
      frame "Apply Network Settings Check" {
        # "If we need to apply static network settings to each target, do so now.\nReboot each target into run mode and wait for it to come back so we know it succeeded.\nOtherwise, reboot each target into run mode but do not bother waiting for it to come back."
        n125 = Unbundle By Name(w440) -> ("Deployment Notifiers"=w428:T1[], "RT Deployment Targets"=w437:T2[], "Target Config. Options"=w438:T4)
        n126 = Unbundle By Name(w438) -> ("Target Config Operation"=w439:T5)
        n127 = Or Array Elements(Boolean array=w426) -> (logical OR=w427:bool)
        n128 = Equal?(x=w439, y=rad_Target_Configuration_Operations."Static Config") -> (x = y?=w443:bool)
        n129 = case shown="True" w443 {
          tunnel: w441 -> [_ w462]
          tunnel: [w449 w461] -> w432
          tunnel: [w453 w460] -> w436
          tunnel: w438 -> [w453 w459]
          tunnel: w437 -> [w452 w458]
          tunnel: [w452 w457] -> w435
          tunnel: w428 -> [w448 w456]
          tunnel: w427 -> [_ w455]
          tunnel: [w448 w454] -> w425
          frame False {
            n130 = Array Size(array=w452) -> (size(s)=w451:i32)
            n131 = Initialize Array(errorcluster {"status"=FALSE, "code"=0, "source"=""} ("error out"), w451) -> (w449:errorcluster[])
          }
          frame True {
            n132 = for {
              tunnel: w462 -> [w471]
              tunnel: [w470] -> w461 mode=indexing
              tunnel: w458 -> [w467] mode=indexing
              shift-right: [w469] -> w460
              shift-left: w459 -> [w468]
              tunnel: [w466] -> w457 mode=indexing
              tunnel: w456 -> [w465] mode=indexing
              tunnel: w455 -> [w464]
              tunnel: [w463] -> w454 mode=indexing
              n133 = case shown="False" w464 {
                tunnel: w471 -> [w480 w488]
                tunnel: [w475 w488] -> w470
                tunnel: [w484 w487] -> w469
                tunnel: w468 -> [w483 w487]
                tunnel: w467 -> [w473 w486]
                tunnel: [w472 w486] -> w466
                tunnel: w465 -> [w474 w485]
                tunnel: [w474 w485] -> w463
                frame False {
                  n134 = Unbundle By Name(w474) -> ("Status"=w481:refnum<notifier>)
                  n135 = Send Notification(notification="Applying deployment network settings...", notifier=w481, error in (no error)=w480) -> (error out=w479:errorcluster)  [unwired: 1 out]
                  n136 = call "rad_Configure Target.vi"("error in (no error)"=w479, "Target settings in"=w473, "Target Config Options in"=w483) -> ("error out"=w476:errorcluster, "Target settings out"=w472:T2, "Target Config Options out"=w484:T4)  [unwired: 6 in]
                  n137 = Unbundle By Name(w474) -> ("Status"=w478:refnum<notifier>)
                  n138 = Send Notification(notification="Network settings applied.", notifier=w478, error in (no error)=w476) -> (error out=w475:errorcluster)  [unwired: 1 out]
                }
                frame True {
                }
              }
            }
          }
        }
        n139 = Bundle By Name(cluster=w440, "RT Deployment Targets"=w435, "Target Config. Options"=w436) -> (w442:T10)
        n140 = call "rad_Deployment Error Handler.vi"("Deployment Notifiers"=w425, "error in (no error)"=w432, "Error Occurred"=w426, "Queue in"=w433) -> ("error out"=w430:errorcluster, "Error Occurred"=w431:bool[], "Queue out"=w429:refnum<queue>)  [unwired: 5 in]
        n141 = Select(t="Exit", s=w443, f="Reboot No Wait") -> (s? t:f=w434:string)
        n142 = Enqueue Element(queue=w429, element=w434, error in (no error)=w430) -> (error out=w446:errorcluster)  [unwired: 1 in, 2 out]
      }
      frame "Reboot No Wait" {
        # "We're done imaging the target, put it back into run mode."
        n143 = Unbundle By Name(w489) -> ("Deployment Notifiers"=w490:T1[], "RT Deployment Targets"=w499:T2[])
        n144 = for {
          tunnel: w499 -> [w502] mode=indexing
          tunnel: w498 -> [w504]
          tunnel: [w503] -> w493 mode=indexing
          tunnel: w491 -> [w501] mode=indexing
          workers-P: _ -> [_]
          n145 = case shown="False" w501 {
            tunnel: w504 -> [w507 w509]
            tunnel: [w506 w509] -> w503
            tunnel: w502 -> [w505 _]
            frame False {
              n146 = call "rad_Reboot (IP) Wrapper.vi"("error in (no error)"=w507, "wait for restart? (F)"=FALSE, "Target settings in"=w505) -> ("error out"=w506:errorcluster)  [unwired: 7 in, 1 out]
            }
            frame True {
            }
          }
        }
        n147 = call "rad_Deployment Error Handler.vi"("Deployment Notifiers"=w490, "error in (no error)"=w493, "Error Occurred"=w491, "Queue in"=w496) -> ("error out"=w492:errorcluster, "Error Occurred"=w494:bool[], "Queue out"=w495:refnum<queue>)  [unwired: 5 in]
        n148 = Enqueue Element(queue=w495, element="Exit" ("Message Name"), error in (no error)=w492) -> (error out=w500:errorcluster)  [unwired: 1 in, 2 out]
      }
      frame "Exit" {
        # "Nothing left to do!"
        n149 = Release Queue(queue=w515, error in (no error)=w516) -> (error out=w514:errorcluster)  [unwired: 1 in, 2 out]
        n150 = Unbundle By Name(w513) -> ("Deployment Notifiers"=w512:T1[])
        n151 = for {
          tunnel: w512 -> [w518] mode=indexing
          tunnel: w511 -> [w517] mode=indexing
          n152 = case shown="False" w517 {
            tunnel: w518 -> [w519 _]
            frame False {
              n153 = Unbundle By Name(w519) -> ("Status"=w520:refnum<notifier>)
              n154 = Send Notification(notification="Deployment Complete!", notifier=w520) -> ()  [unwired: 1 in, 2 out]
            }
            frame True {
            }
          }
        }
      }
    }
  }
  "Error Occurred" <- w5
  n155 = Unbundle By Name(w9) -> ("Target Config. Options"=→"Target Config Options out":T4)
